vi "FICHEROS.vi"() -> ()   [LabVIEW 2020]
uses:
  <vilib>/ErrorRing/Error Ring.xnode
panel:
  in  "Combo Box":string(combo)
  in  "Nombre del archivo":string
  in  "base path":path
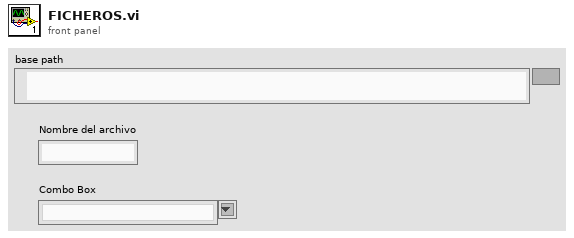
[diagram p1: front panel]
types:
  T1 = enum16{"open", "replace", "create", "open or create", "replace or create", "replace or create with confirmation"}
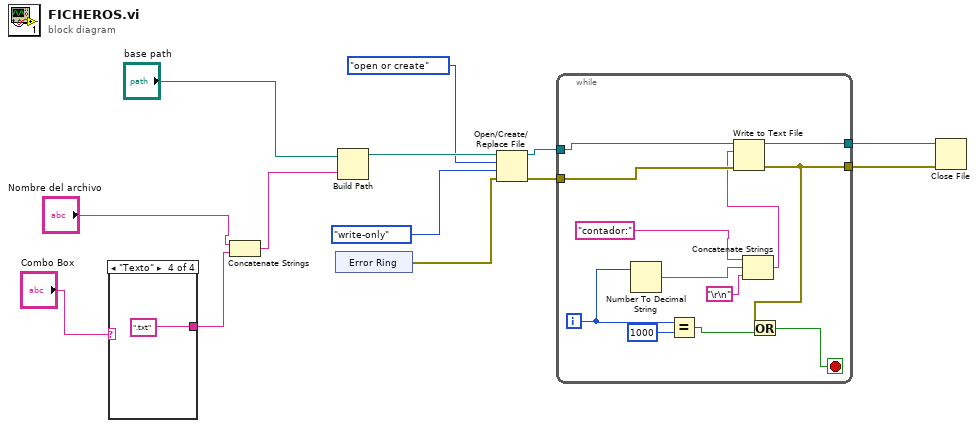
[diagram p0: block diagram]
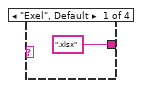
[diagram p2: hidden frame]
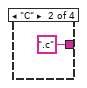
[diagram p3: hidden frame]
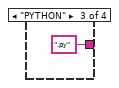
[diagram p4: hidden frame]
diagram:
  n1 = case shown="\"Texto\"" "Combo Box" {
    tunnel: [".xlsx" ".c" ".py" ".txt"] -> w10
    frame "Exel", Default {
    }
    frame "C" {
    }
    frame "PYTHON" {
    }
    frame "Texto" {
    }
  }
  n2 = Concatenate Strings("Nombre del archivo", w10) -> (w9:string)
  n3 = xnode "Error Ring"() -> ("error out"=w5:errorcluster)
  n4 = Build Path(base path="base path", name or relative path=w9) -> (appended path=w8:path)
  n5 = Open/Create/Replace File(file path (use dialog)=w8, error in=w5, operation (0:open)=T1."open or create", access (0:read/write)=enum16{"read/write", "read-only", "write-only"}."write-only") -> (refnum out=w4:refnum<file>, error out=w3:errorcluster)  [unwired: 2 in, 1 out]
  n6 = while {
    tunnel: w4 -> [w26]
    tunnel: w3 -> [w25]
    tunnel: [w24] -> w2
    tunnel: [w19] -> w1
    i -> [w22]
    stop <- w18 stop-if-true
    n7 = Number To Decimal String(number=w22) -> (decimal integer string=w28:string)  [unwired: 1 in]
    n8 = Equal?(x=w22, y=1000) -> (x = y?=w20:bool)
    n9 = Concatenate Strings("contador:", w28, "\r\n") -> (w23:string)
    n10 = Write to Text File(file (use dialog)=w26, text=w23, error in=w25) -> (refnum out=w24:refnum<file>, error out=w19:errorcluster)  [unwired: 1 in, 1 out]
    n11 = Or(x=w19, y=w20) -> (x .or. y?=w18:bool)
  }
  n12 = Close File(refnum=w2, error in=w1) -> ()  [unwired: 2 out]
